vi "Unloading_Section_To_Run_Check.vi"(7 "Cluster DATA IN":T1, 8 "error in (no error)":errorcluster) -> (0 "error out":errorcluster, 2 "FULLY UNLOADED FOUND ?":bool, 5 "Cluster DATA OUT":T1)   [LabVIEW 2017]
uses:
  Controls/Unload_Cyc_Data.ctl
  <vilib>/Utility/file.llb/Read Delimited Spreadsheet (string).vi
panel:
  # "UNLOAD"
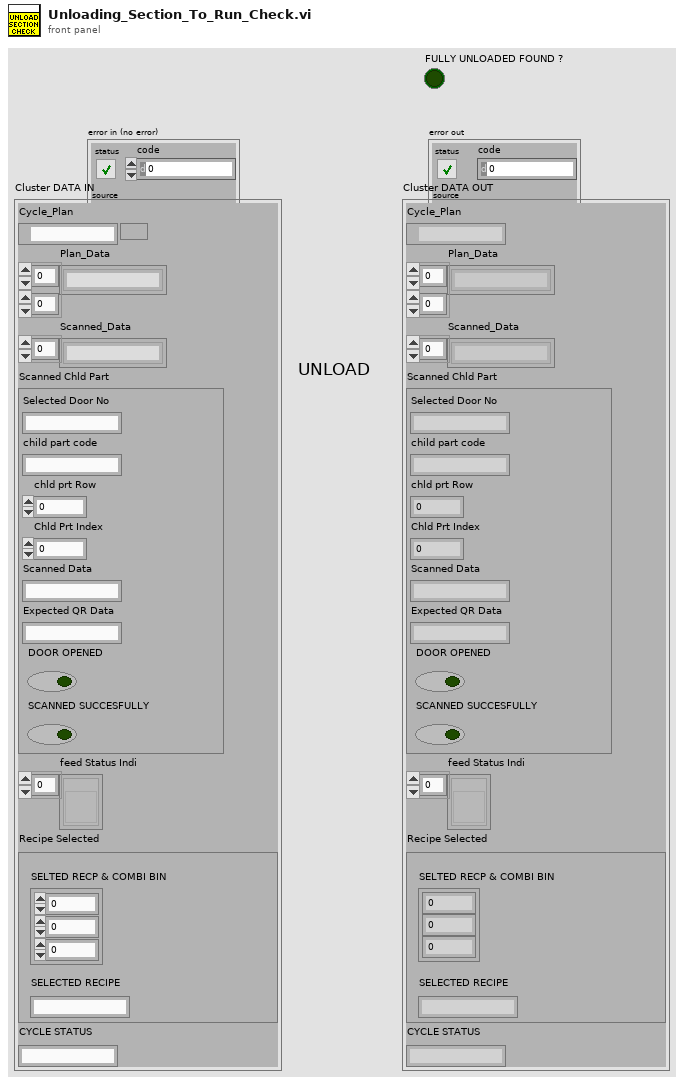
[diagram p1: front panel]
types:
  T1 = typedef "Unload_Cyc_Data.ctl" = cluster{"Cycle_Plan":path, "Plan_Data":string[][], "Scanned_Data":string[], "Scanned Chld Part":cluster{"Selected Door No":string, "child part code":string, "chld prt Row":i32, "Chld Prt Index":i32, "Scanned Data":string, "Expected QR Data":string, "DOOR OPENED":bool, "SCANNED SUCCESFULLY":bool}, "feed Status Indi":refnum<vi>[], "Recipe Selected":cluster{"SELTED RECP & COMBI BIN":cluster{"RECIPE INDEX":i32, "COMBI BIN":i32, "Section row no.":i32}, "SELECTED RECIPE":string}, "CYCLE STATUS":string}
  T2 = cluster{"RECIPE INDEX":i32, "COMBI BIN":i32, "Section row no.":i32}
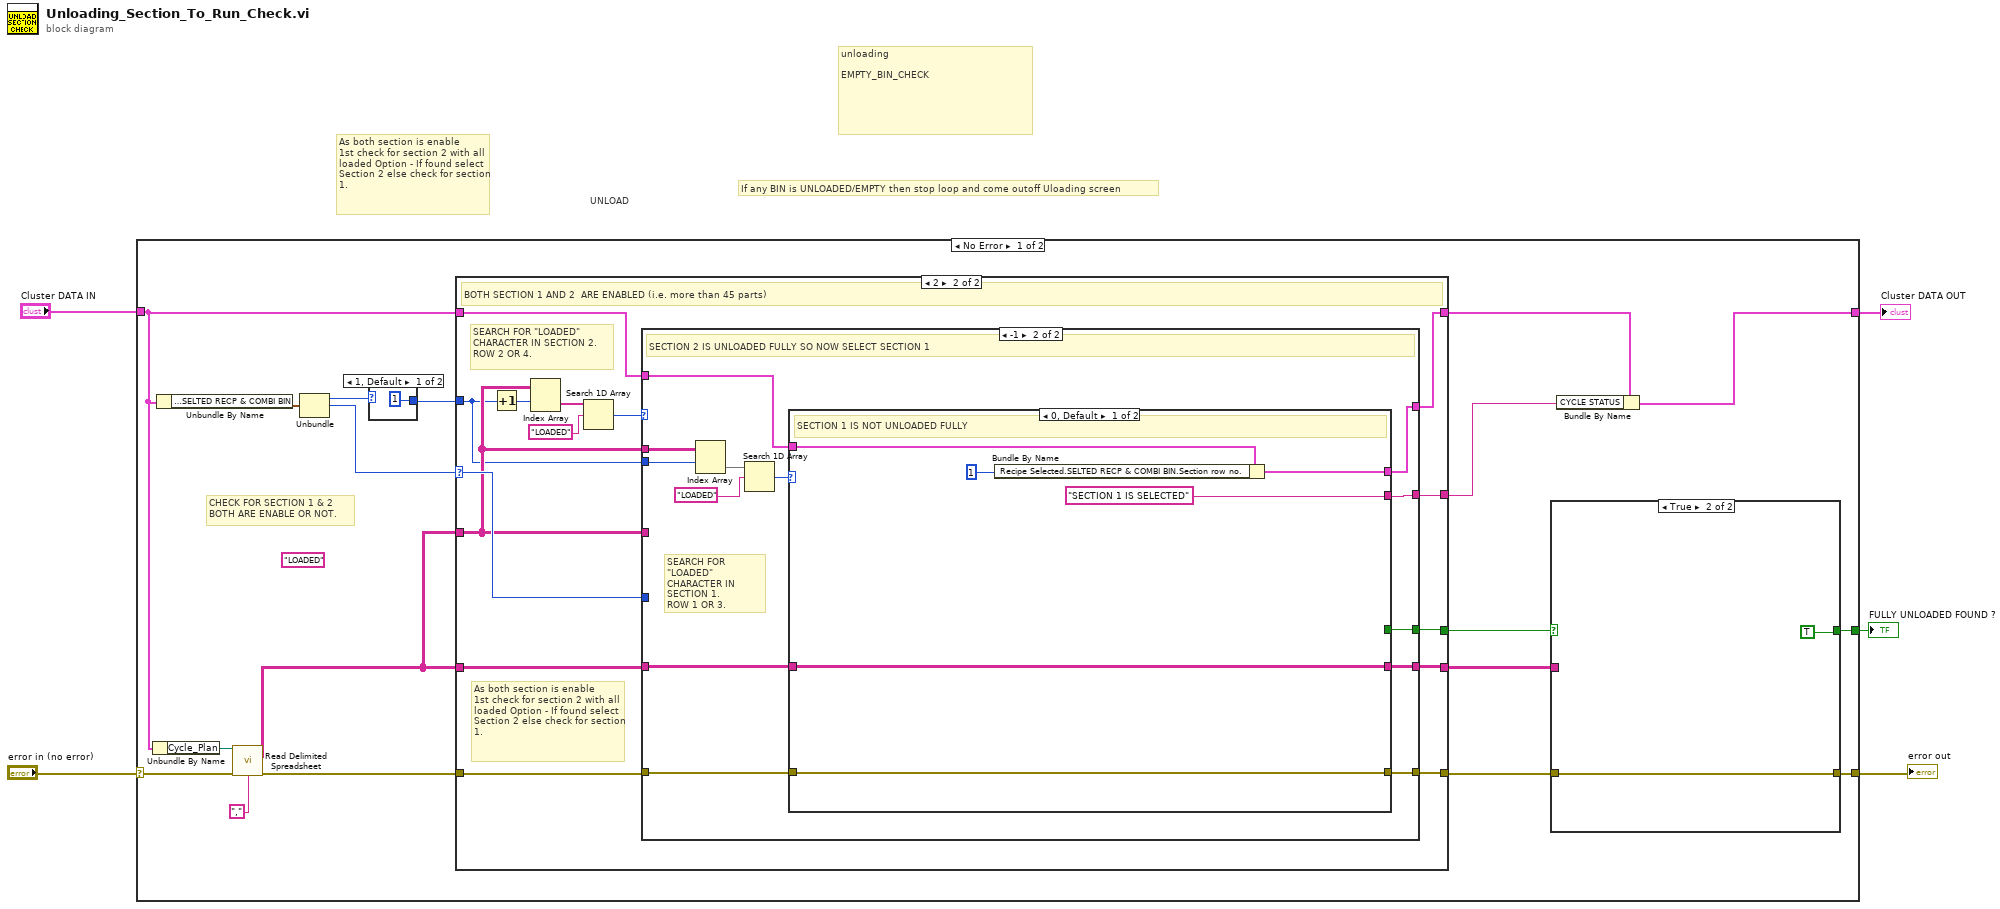
[diagram p0: block diagram]
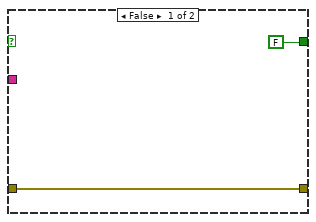
[diagram p2: hidden frame]
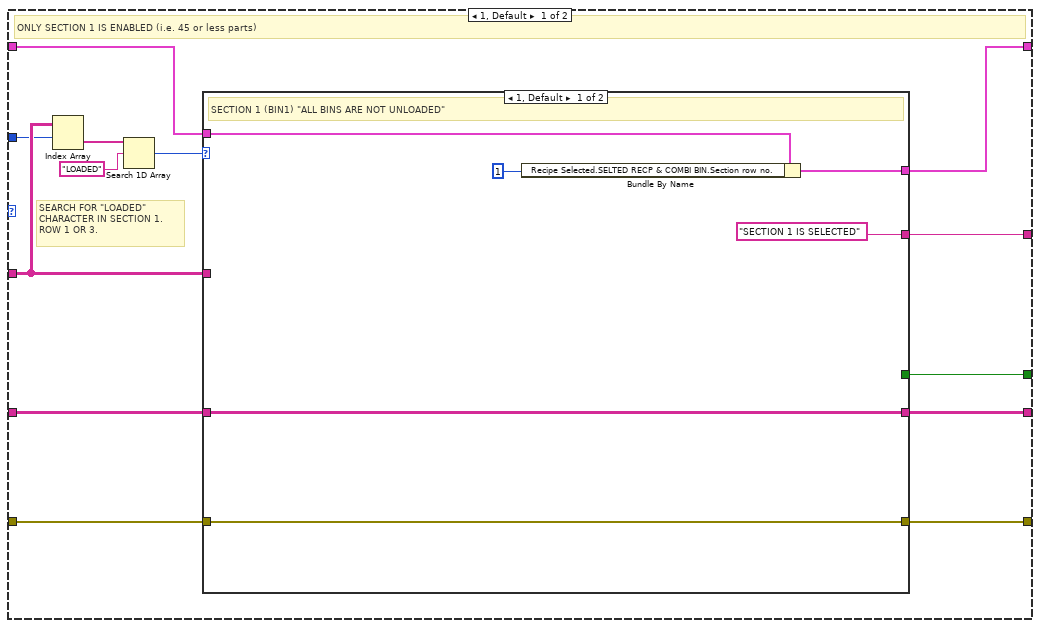
[diagram p3: hidden frame]
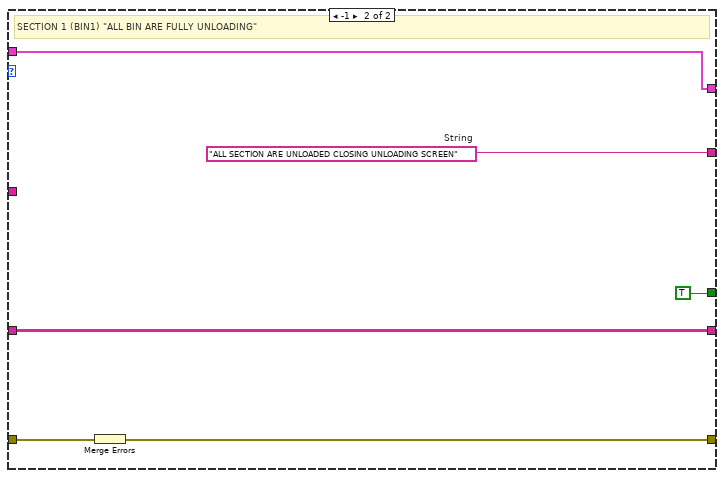
[diagram p4: hidden frame]
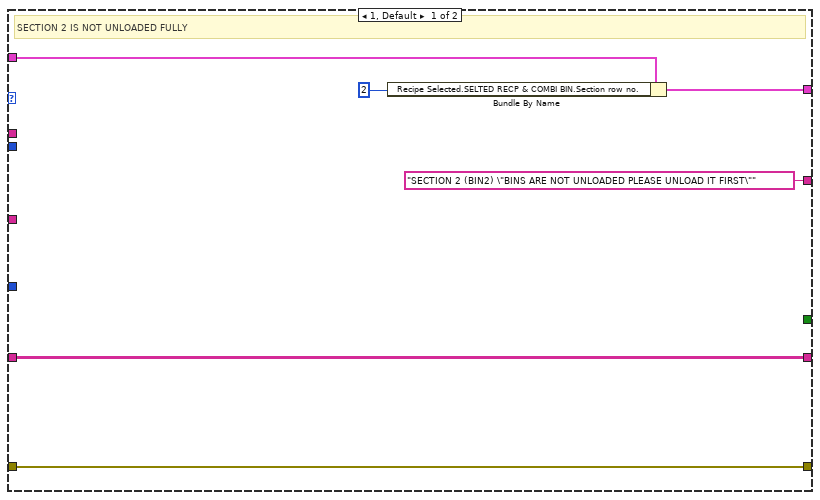
[diagram p5: hidden frame]
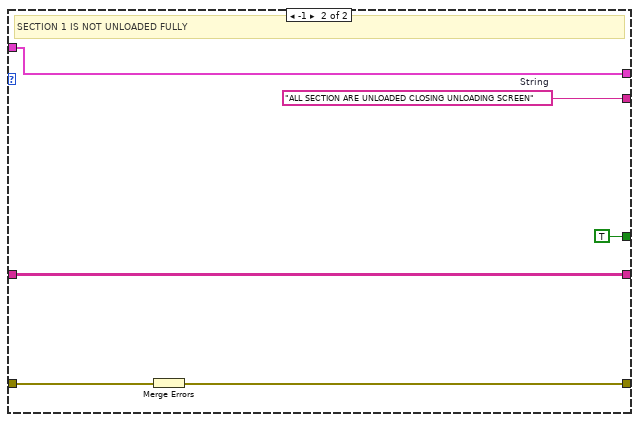
[diagram p6: hidden frame]
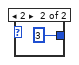
[diagram p7: hidden frame]
diagram:
  # "As both section is enable\n1st check for section 2 with all loaded Option - If found select Section 2 else check for section 1."
  # "UNLOAD"
  # "If any BIN is UNLOADED/EMPTY then stop loop and come outoff Uloading screen"
  # "unloading\n\nEMPTY_BIN_CHECK"
  n1 = case shown="No Error" "error in (no error)" {
    selector: "error in (no error)" -> [w20 w102]
    tunnel: [w12 w102] -> w4
    tunnel: [w7 w101] -> w2
    tunnel: "Cluster DATA IN" -> [w16 w101]
    tunnel: [w9 _] -> w1
    frame No Error {
      (unwired) "LOADED"
      # "CHECK FOR SECTION 1 & 2\nBOTH ARE ENABLE OR NOT."
      n2 = Unbundle By Name(w16) -> ("Cycle_Plan"=w21:path)
      n3 = Unbundle By Name(w16) -> ("Recipe Selected.SELTED RECP & COMBI BIN"=w18:T2)
      n4 = call-poly <vilib>:"Read Delimited Spreadsheet.vi"("file path (dialog if empty)"=w21, "error in (no error)"=w20, "delimiter (\\t)"=",") -> ("all rows"=w14:string[][], "error out"=w19:errorcluster)  [unwired: 7 in, 4 out]
      n5 = Unbundle(w18) -> ("RECIPE INDEX"=w17:i32, "COMBI BIN"=w13:i32)  [unwired: 1 out]
      n6 = case shown="1, Default" w17 {
        tunnel: [1 3] -> w15
        frame 1, Default {
        }
        frame 2 {
        }
      }
      n7 = case shown="2" w13 {
        selector: w13 -> [_ w59]
        tunnel: [w39 w65] -> w23
        tunnel: w19 -> [w40 w66]
        tunnel: [w28 w53] -> w8
        tunnel: w16 -> [w29 w54]
        tunnel: w14 -> [w36 w57]
        tunnel: w15 -> [w33 w56]
        tunnel: w14 -> [w38 w67]
        tunnel: [w37 w64] -> w10
        tunnel: [w35 w63] -> w11
        tunnel: [w34 w62] -> w6
        frame 1, Default {
          # "SEARCH FOR \"LOADED\"\nCHARACTER IN SECTION 1.\nROW 1 OR 3."
          # "ONLY SECTION 1 IS ENABLED (i.e. 45 or less parts)"
          n8 = Index Array(array=w36, index (row)=w33) -> (element=w32:string[])  [unwired: 1 in]
          n9 = Search 1D Array(1D array=w32, element="LOADED") -> (index of element=w30:i32)  [unwired: 1 in]
          n10 = case shown="1, Default" w30 {
            tunnel: w40 -> [w46 w52]
            tunnel: [w46 w51] -> w39
            tunnel: w38 -> [w45 w50]
            tunnel: [w45 w50] -> w37
            tunnel: w36 -> [_ _]
            tunnel: [_ TRUE] -> w35
            tunnel: ["SECTION 1 IS SELECTED" w48] -> w34
            tunnel: w29 -> [w42 w47]
            tunnel: [w41 w47] -> w28
            frame 1, Default {
              # "SECTION 1 (BIN1) \"ALL BINS ARE NOT UNLOADED\""
              n11 = Bundle By Name(cluster=w42, "Recipe Selected.SELTED RECP & COMBI BIN.Section row no."=1) -> (w41:T1)
            }
            frame -1 {
              w48 = "ALL SECTION ARE UNLOADED CLOSING UNLOADING SCREEN"  # String
              # "SECTION 1 (BIN1) \"ALL BIN ARE FULLY UNLOADING\""
              n12 = Merge Errors(w52) -> (w51:errorcluster)
            }
          }
        }
        frame 2 {
          # "As both section is enable\n1st check for section 2 with all loaded Option - If found select Section 2 else check for section 1."
          # "SEARCH FOR \"LOADED\"\nCHARACTER IN SECTION 2.\nROW 2 OR 4."
          # "BOTH SECTION 1 AND 2  ARE ENABLED (i.e. more than 45 parts)"
          n13 = Increment(x=w56) -> (x+1=w55:i32)
          n14 = Index Array(array=w57, index (row)=w55) -> (element=w61:string[])  [unwired: 1 in]
          n15 = Search 1D Array(1D array=w61, element="LOADED") -> (index of element=w58:i32)  [unwired: 1 in]
          n16 = case shown="-1" w58 {
            tunnel: [w73 w85] -> w65
            tunnel: w66 -> [w73 w86]
            tunnel: [w72 w84] -> w64
            tunnel: w67 -> [w72 w83]
            tunnel: w57 -> [_ _]
            tunnel: w59 -> [_ _]
            tunnel: [_ w82] -> w63
            tunnel: ["SECTION 2 (BIN2) \"BINS ARE NOT UNLOADED PLEASE UNLOAD IT FIRST\"" w78] -> w62
            tunnel: w57 -> [_ w81]
            tunnel: w56 -> [_ w76]
            tunnel: w54 -> [w70 w75]
            tunnel: [w68 w74] -> w53
            frame 1, Default {
              # "SECTION 2 IS NOT UNLOADED FULLY"
              n17 = Bundle By Name(cluster=w70, "Recipe Selected.SELTED RECP & COMBI BIN.Section row no."=2) -> (w68:T1)
            }
            frame -1 {
              # "SEARCH FOR \"LOADED\"\nCHARACTER IN SECTION 1.\nROW 1 OR 3."
              # "SECTION 2 IS UNLOADED FULLY SO NOW SELECT SECTION 1"
              n18 = Index Array(array=w81, index (row)=w76) -> (element=w80:string[])  [unwired: 1 in]
              n19 = Search 1D Array(1D array=w80, element="LOADED") -> (index of element=w77:i32)  [unwired: 1 in]
              n20 = case shown="0, Default" w77 {
                tunnel: w86 -> [w92 w98]
                tunnel: [w92 w97] -> w85
                tunnel: [w91 w96] -> w84
                tunnel: w83 -> [w91 w96]
                tunnel: [_ TRUE] -> w82
                tunnel: ["SECTION 1 IS SELECTED" w95] -> w78
                tunnel: w75 -> [w88 w93]
                tunnel: [w87 w93] -> w74
                frame 0, Default {
                  # "SECTION 1 IS NOT UNLOADED FULLY"
                  n21 = Bundle By Name(cluster=w88, "Recipe Selected.SELTED RECP & COMBI BIN.Section row no."=1) -> (w87:T1)
                }
                frame -1 {
                  w95 = "ALL SECTION ARE UNLOADED CLOSING UNLOADING SCREEN"  # String
                  # "SECTION 1 IS NOT UNLOADED FULLY"
                  n22 = Merge Errors(w98) -> (w97:errorcluster)
                }
              }
            }
          }
        }
      }
      n23 = case shown="True" w11 {
        tunnel: w23 -> [w25 w27]
        tunnel: [w25 w27] -> w12
        tunnel: w10 -> [_ _]
        tunnel: [FALSE TRUE] -> w9
        frame False {
        }
        frame True {
        }
      }
      n24 = Bundle By Name(cluster=w8, "CYCLE STATUS"=w6) -> (w7:T1)
    }
    frame Error {
    }
  }
  "error out" <- w4
  "Cluster DATA OUT" <- w2
  "FULLY UNLOADED FOUND ?" <- w1
